vi "Read Data.vi"(8 "error in (no error)":errorcluster, 11 "Double in":refnum<class "Double.lvclass">) -> (0 "error out":errorcluster, 2 "Data":dbl, 3 "Double out":refnum<class "Double.lvclass">)   [LabVIEW 2012, in "Base Data Class.lvlib" / "Double.lvclass"]
uses:
  Double.lvclass
  Double.lvclass/Double.ctl
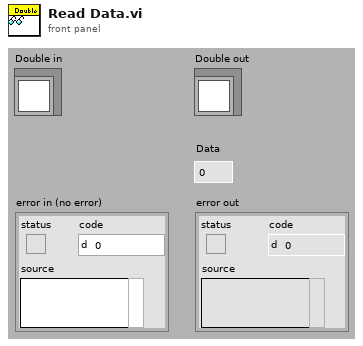
[diagram p1: front panel]
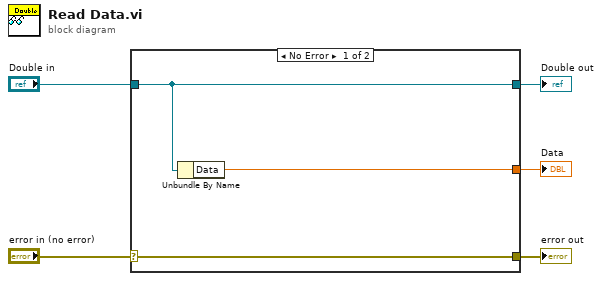
[diagram p0: block diagram]
diagram:
  n1 = case shown="No Error" "error in (no error)" {
    selector: "error in (no error)" -> [w8 w9]
    tunnel: [w8 w9] -> w4
    tunnel: [w7 w10] -> w2
    tunnel: "Double in" -> [w7 w10]
    tunnel: [w6 _] -> w1
    frame No Error {
      n2 = Unbundle By Name(w7) -> ("Data"=w6:dbl)
    }
    frame Error {
    }
  }
  "error out" <- w4
  "Double out" <- w2
  "Data" <- w1
